vi "Check if Backup Already Exists.vi"(6 "Error Message in":string, 8 "Error In":errorcluster, 10 "Full App Name":string="PC Interface.exe", 11 "Local Version Array":i32[](array[numeric])) -> (0 "Error Out":errorcluster, 2 "File Exists":bool, 3 "Filename":string, 4 "Error Message out":string)   [LabVIEW 2019]
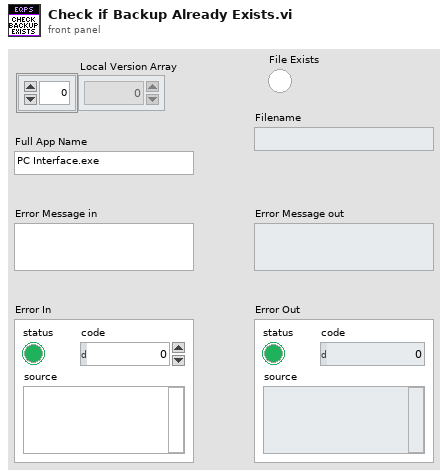
[diagram p1: front panel]
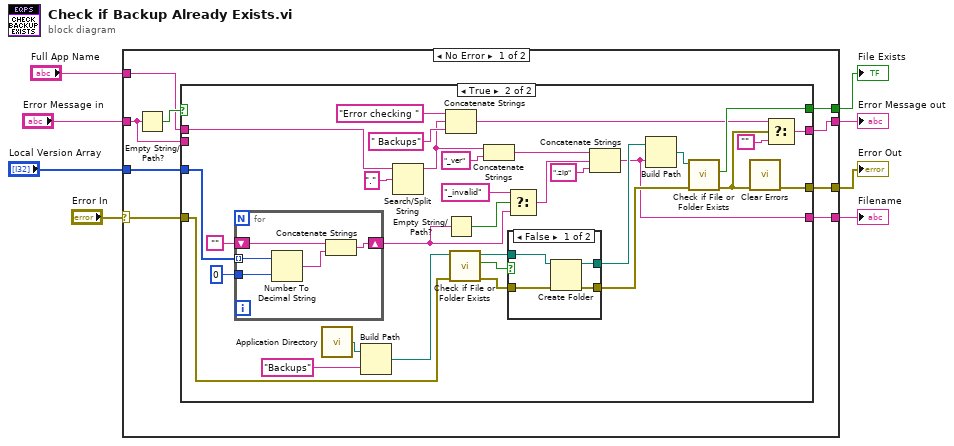
[diagram p0: block diagram]
diagram:
  n1 = case shown="No Error" "Error In" {
    selector: "Error In" -> [w13 w64]
    tunnel: [w14 w64] -> w7
    tunnel: [w16 w63] -> w6
    tunnel: "Error Message in" -> [w15 w63]
    tunnel: "Local Version Array" -> [w12 _]
    tunnel: [w11 _] -> w3
    tunnel: [w10 _] -> w2
    tunnel: "Full App Name" -> [w9 _]
    frame No Error {
      n2 = Empty String/Path?(string/path=w15) -> (empty?=w17:bool)
      n3 = case shown="True" w17 {
        tunnel: [w19 w37] -> w16
        tunnel: w15 -> [w19 _]
        tunnel: [w18 w40] -> w14
        tunnel: w13 -> [w18 w49]
        tunnel: w12 -> [_ w31]
        tunnel: [_ w36] -> w11
        tunnel: [_ w35] -> w10
        tunnel: w9 -> [_ w27]
        frame False {
        }
        frame True {
          n4 = for {
            tunnel: w31 -> [w56] mode=indexing
            tunnel: i16 0 ("width (-)") -> [w55]
            shift-right: [w52] -> w28
            shift-left: "" -> [w53]
            n5 = Number To Decimal String(number=w56, width (-)=w55) -> (decimal integer string=w54:string)
            n6 = Concatenate Strings(w53, w54) -> (w52:string)
          }
          n7 = call <vilib>:"Application Directory.vi"() -> ("Application Directory"=w51:path)
          n8 = Build Path(base path=w51, name or relative path="Backups") -> (appended path=w48:path)
          n9 = Search/Split String(string=w27, search string/char (-)=".") -> (substring before match=w22:string)  [unwired: 1 in, 2 out]
          n10 = Concatenate Strings("Error checking ", w22, " Backups") -> (w20:string)
          n11 = Empty String/Path?(string/path=w28) -> (empty?=w34:bool)
          n12 = call <vilib>:"Check if File or Folder Exists.vi"("error in (no error)"=w49, "path"=w48) -> ("error out"=w45:errorcluster, "file or folder exists?"=w47:bool, "dup path"=w46:path)  [unwired: 7 in]
          n13 = Concatenate Strings(w22, "_ver") -> (w24:string)
          n14 = Select(t="_invalid", s=w34, f=w28) -> (s? t:f=w32:string)
          n15 = case shown="False" w47 {
            tunnel: w46 -> [w59 w62]
            tunnel: w45 -> [w60 w61]
            tunnel: [w58 w62] -> w42
            tunnel: [w57 w61] -> w43
            frame False {
              n16 = Create Folder(path (use dialog)=w59, error in=w60) -> (created path=w58:path, error out=w57:errorcluster)  [unwired: 1 in, 1 out]
            }
            frame True {
            }
          }
          n17 = Concatenate Strings(w24, w32, ".zip") -> (w35:string)
          n18 = Build Path(base path=w42, name or relative path=w35) -> (appended path=w41:path)
          n19 = call <vilib>:"Check if File or Folder Exists.vi"("error in (no error)"=w43, "path"=w41) -> ("error out"=w39:errorcluster, "file or folder exists?"=w36:bool)  [unwired: 7 in, 1 out]
          n20 = call <vilib>:"Clear Errors.vi"("error in (no error)"=w39) -> ("error out"=w40:errorcluster)  [unwired: 5 in, 1 out]
          n21 = Select(t=w20, s=w39, f="") -> (s? t:f=w37:string)
        }
      }
    }
    frame Error {
    }
  }
  "Error Out" <- w7
  "Error Message out" <- w6
  "File Exists" <- w3
  "Filename" <- w2
